vi "Check Simulator.vi"(7 "Module Name":string, 8 "error in (no error)":errorcluster) -> (0 "error out":errorcluster, 1 "Arrived?":bool, 2 "Current Position":dbl)   [LabVIEW 2019, in "ADLINK Motion Card.lvlib"]
uses:
  ADLINK Motion Card.lvlib
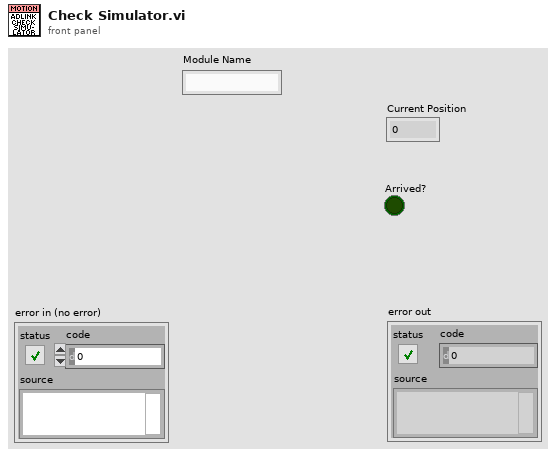
[diagram p1: front panel]
types:
  T1 = typedef "ADLINK Motion Card.lvlib/SEQ Data.ctl" = cluster{"Current Position":dbl, "Target Position":dbl, "Velocity":dbl, "Acceleration":dbl, "Arrived?":bool, "data value reference":refnum<data-value>, "VI Refnum":refnum<vi>}
  T2 = cluster{"Current Position":dbl, "Target Position":dbl, "Velocity":dbl, "Acceleration":dbl, "Arrived?":bool}
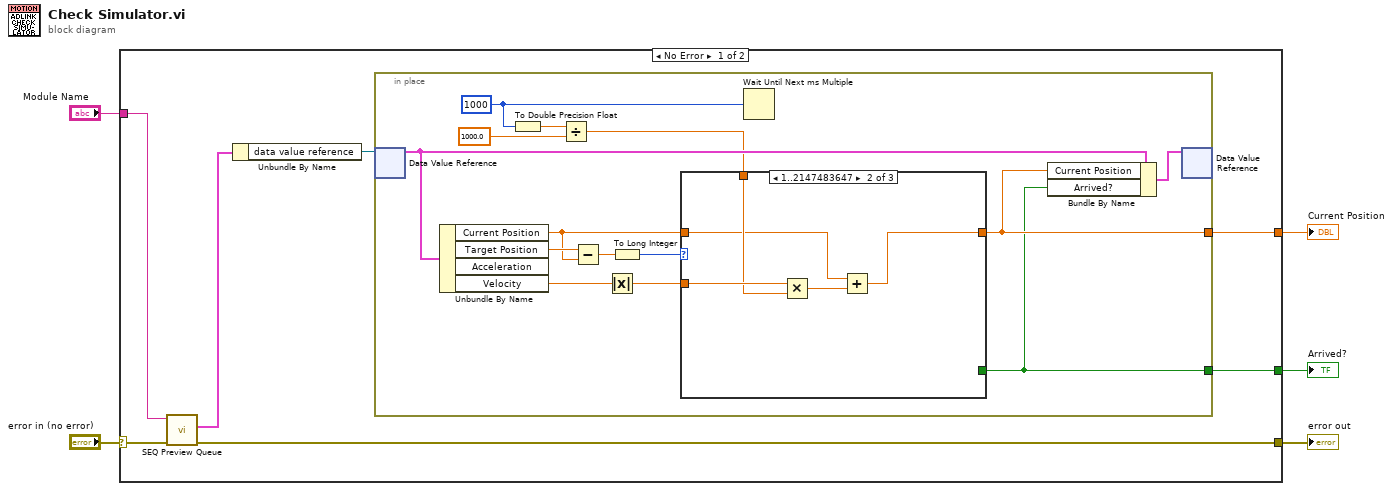
[diagram p0: block diagram]
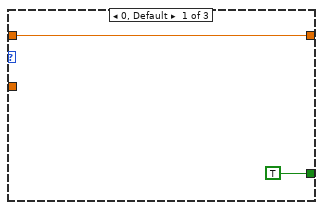
[diagram p2: hidden frame]
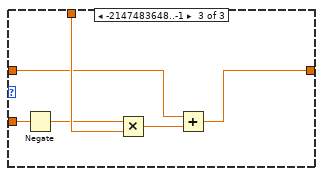
[diagram p3: hidden frame]
diagram:
  n1 = case shown="No Error" "error in (no error)" {
    selector: "error in (no error)" -> [w11 w40]
    tunnel: [w8 w40] -> w5
    tunnel: "Module Name" -> [w12 _]
    tunnel: [w7 _] -> w2
    tunnel: [w6 _] -> w1
    frame No Error {
      n2 = call "SEQ Preview Queue.vi"("error in (no error)"=w11, "Queue Name"=w12) -> ("error out"=w8:errorcluster, "Setting"=w10:T1)  [unwired: 8 in]
      n3 = Unbundle By Name(w10) -> ("data value reference"=w9:refnum<data-value>)
      n4 = in-place {
        in-place-border: [w14] -> w7
        in-place-border: [w13] -> w6
        w20 = u32 1000 ("millisecond multiple")
        n5 = in-place-dvr #1(w9) -> (w26:T2)  [unwired: 1 out]
        n6 = Unbundle By Name(w26) -> ("Current Position"=w21:dbl, "Target Position"=w24:dbl, "Velocity"=w15:dbl)  [unwired: 1 out]
        n7 = To Double Precision Float(number=w20) -> (double precision float=w19:dbl)
        n8 = Divide(x=w19, y=1000.0) -> (x/y=w17:dbl)
        n9 = Subtract(x=w24, y=w21) -> (x-y=w23:dbl)
        n10 = Absolute Value(x=w15) -> (abs(x)=w16:dbl)
        n11 = To Long Integer(number=w23) -> (32bit integer=w22:i32)
        n12 = case shown="1..2147483647" w22 {
          tunnel: w21 -> [w28 w30 w36]
          tunnel: [w28 w29 w35] -> w14
          tunnel: [TRUE _ _] -> w13
          tunnel: w16 -> [_ w33 w39]
          tunnel: w17 -> [_ w32 w38]
          frame 0, Default {
          }
          frame 1..2147483647 {
            n13 = Multiply(x=w33, y=w32) -> (x*y=w31:dbl)
            n14 = Add(x=w30, y=w31) -> (x+y=w29:dbl)
          }
          frame -2147483648..-1 {
            n15 = Negate(x=w39) -> (-x=w34:dbl)
            n16 = Multiply(x=w34, y=w38) -> (x*y=w37:dbl)
            n17 = Add(x=w36, y=w37) -> (x+y=w35:dbl)
          }
        }
        n18 = Wait Until Next ms Multiple(millisecond multiple=w20) -> ()  [unwired: 1 out]
        n19 = Bundle By Name(cluster=w26, "Current Position"=w14, "Arrived?"=w13) -> (w25:T2)
        n20 = in-place-dvr #1(w25) -> ()  [unwired: 2 out]
      }
    }
    frame Error {
    }
  }
  "error out" <- w5
  "Current Position" <- w2
  "Arrived?" <- w1
